vi "Write My Data to CSV.vi"(4 "Data":T1(array[cluster]), 5 "Comment":string, 7 "Time Stamp":timestamp, 8 "error in":errorcluster, 11 "file path":path) -> (0 "error out":errorcluster)   [LabVIEW 2014]
panel:
  out "concatenated string":string
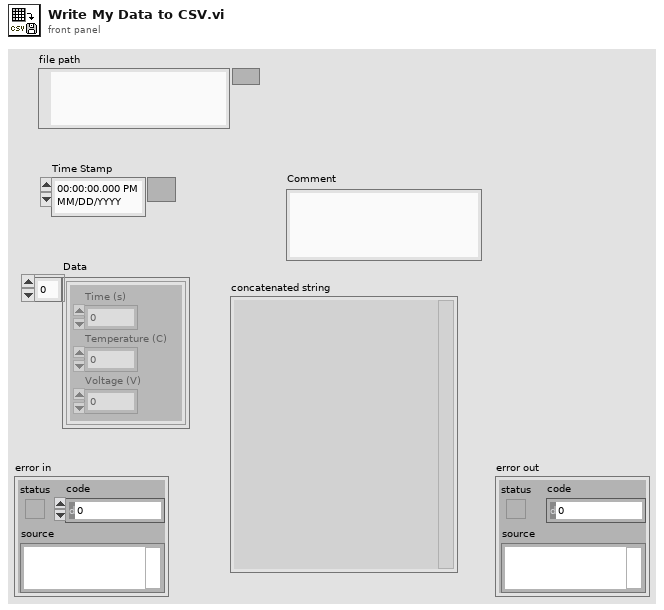
[diagram p1: front panel]
types:
  T1 = cluster{"Time (s)":dbl, "Temperature (C)":dbl, "Voltage (V)":dbl}[]
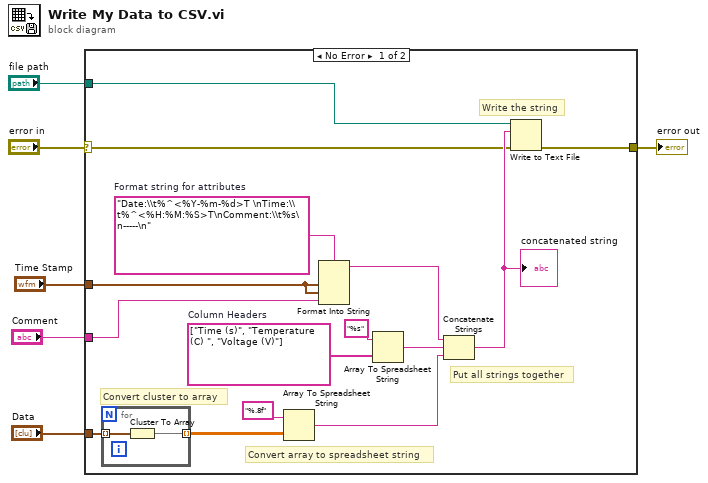
[diagram p0: block diagram]
diagram:
  n1 = case shown="No Error" "error in" {
    selector: "error in" -> [w11 w24]
    tunnel: "Data" -> [w15 _]
    tunnel: [w12 w24] -> w6
    tunnel: "file path" -> [w13 _]
    tunnel: "Time Stamp" -> [w9 _]
    tunnel: "Comment" -> [w8 _]
    frame No Error {
      w10 = "Date:\\t%^<%Y-%m-%d>T \nTime:\\t%^<%H:%M:%S>T\nComment:\\t%s\n-----\n"  # Format string for attributes
      w20 = string[] ["Time (s)", "Temperature (C) ", "Voltage (V)"]  # Column Headers
      # "Write the string"
      # "Put all strings together"
      # "Convert array to spreadsheet string"
      # "Convert cluster to array"
      n2 = for {
        tunnel: w15 -> [w23] mode=indexing
        tunnel: [w22] -> w14 mode=indexing
        n3 = Cluster To Array(cluster=w23) -> (array=w22:dbl[])
      }
      n4 = Array To Spreadsheet String(array=w14, 3:"%.8f" ("format string")) -> (spreadsheet string=w18:string)  [unwired: 1 in]
      n5 = Format Into String(format string=w10, w9, w9, w8) -> (resulting string=w7:string)  [unwired: 2 in, 1 out]
      n6 = Array To Spreadsheet String(array=w20, 3:"%s" ("format string")) -> (spreadsheet string=w19:string)  [unwired: 1 in]
      n7 = Concatenate Strings(w7, w19, w18) -> (w17:string)
      "concatenated string" <- w17
      n8 = Write to Text File(file (use dialog)=w13, text=w17, error in=w11) -> (error out=w12:errorcluster)  [unwired: 1 in, 2 out]
    }
    frame Error {
      # "Wire previous error through"
    }
  }
  "error out" <- w6
